vi "NI-Test.vi"() -> ()   [LabVIEW 2017]
uses:
  <vilib>/Utility/config.llb/Read Key (String).vi
  <vilib>/Utility/config.llb/NI_LVConfig.lvlib
panel:
  out "Press":dbl[][](array[numeric])
  out "FT":dbl[][](array[numeric])
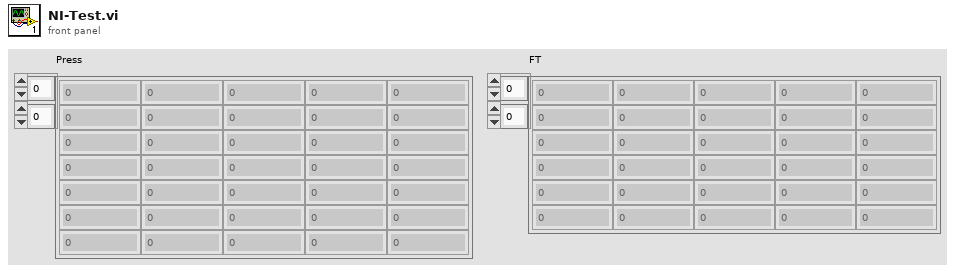
[diagram p1: front panel]
types:
  T1 = typedef "NI_LVConfig.lvlib/Config Data RefNum.ctl" = refnum<k1>
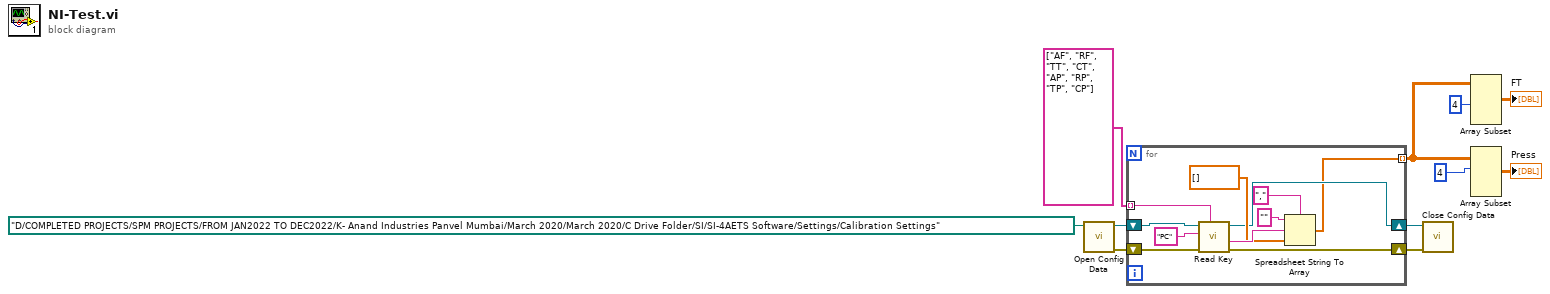
[diagram p0: block diagram]
diagram:
  n1 = call <vilib>:"Open Config Data.vi"("configuration file path"=path "D:/COMPLETED PROJECTS/SPM PROJECTS/FROM JAN2022 TO DEC2022/K- Anand Industries Panvel Mumbai/March 2020/March 2020/C Drive Folder/SI/SI-4AETS Software/Settings/Calibration Settings") -> ("error out"=w9:errorcluster, "refnum"=w8:T1)  [unwired: 8 in, 1 out]
  n2 = for {
    shift-right: [w18] -> w11
    shift-left: w9 -> [w15]
    shift-right: [w17] -> w10
    shift-left: w8 -> [w14]
    tunnel: string[] ["AF", "RF", "TT", "CT", "AP", "RP", "TP", "CP"] -> [w13] mode=indexing
    tunnel: [w12] -> w6 mode=indexing
    n3 = call-poly <vilib>:"Read Key.vi"("section"=w13, "error in (no error)"=w15, "key"="PC" ("c Tabl"), "refnum"=w14) -> ("error out"=w18:errorcluster, "value"=w22:string, "refnum out"=w17:T1)  [unwired: 4 in, 1 out]
    n4 = Spreadsheet String To Array(delimiter (Tab)=",", format string="", spreadsheet string=w22, array type (2D Dbl)=dbl[] []) -> (array=w12:dbl[])
  }
  n5 = call <vilib>:"Close Config Data.vi"("error in (no error)"=w11, "refnum"=w10) -> ()  [unwired: 8 in, 2 out]
  n6 = Array Subset(array=w6, length (row)=4 ("length")) -> (→"FT":dbl[][])  [unwired: 3 in]
  n7 = Array Subset(array=w6, index (row)=4 ("length")) -> (→"Press":dbl[][])  [unwired: 3 in]
